vi "Write Bln_Continuous.vi"(8 "error in (no error)":errorcluster, 10 "Continuous?":bool, 11 "Bobcat 640 in":refnum<class "Bobcat 640.lvclass">) -> (0 "error out":errorcluster, 3 "Bobcat 640 out":refnum<class "Bobcat 640.lvclass">)   [LabVIEW 2018, in "Bobcat 640.lvlib" / "Bobcat 640.lvclass"]
uses:
  Bobcat 640.lvclass
  Bobcat 640.lvclass/Bobcat 640.ctl
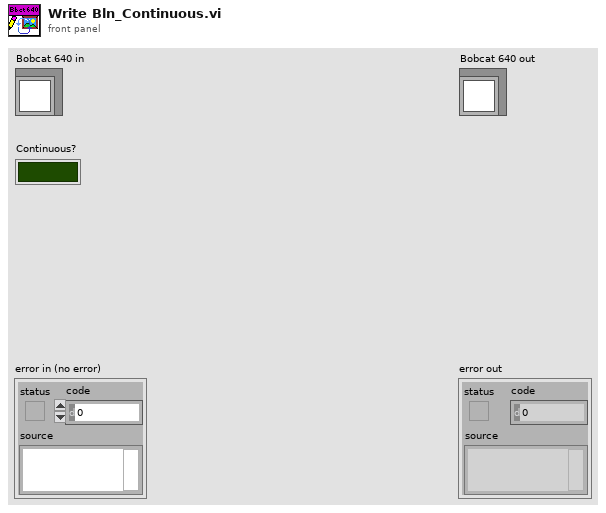
[diagram p1: front panel]
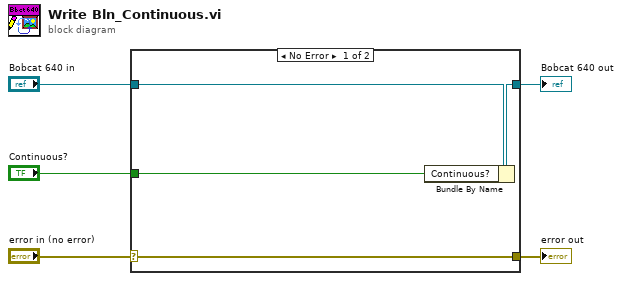
[diagram p0: block diagram]
diagram:
  n1 = case shown="No Error" "error in (no error)" {
    selector: "error in (no error)" -> [w9 w10]
    tunnel: [w9 w10] -> w4
    tunnel: [w7 w11] -> w2
    tunnel: "Bobcat 640 in" -> [w8 w11]
    tunnel: "Continuous?" -> [w6 _]
    frame No Error {
      n2 = Bundle By Name(cluster=w8, "Continuous?"=w6) -> (w7:refnum<class "Bobcat 640.lvclass">)
    }
    frame Error {
    }
  }
  "error out" <- w4
  "Bobcat 640 out" <- w2
